vi "Paths to Commands.vi"(5 "Offset":cluster{"X Offset":dbl, "Y Offset":dbl}, 7 "Scaling":T1={"X Scaling (%)"=100.0, "Y Scaling (%)"=100.0}, 8 "error in (no error)":errorcluster, 10 "Path Properties":T3(array[cluster])=[{"Speed"=100.0, "Direction"=0, "Orientation (For Filled)"=enum."Vertical", "Max Spacing Between\nLines (For Filled)"=0.05, "Start and End Voltage"={"End Voltage"=0.0, "Start Voltage"=0.0}}, {"Speed"=100.0, "Direction"=0, "Orientation (For Filled)"=enum."Vertical", "Max Spacing Between\nLines (For Filled)"=0.05, "Start and End Voltage"={"End Voltage"=0.0, "Start Voltage"=0.0}}, {"Speed"=100.0, "Direction"=0, "Orientation (For Filled)"=enum."Vertical", "Max Spacing Between\nLines (For Filled)"=0.05, "Start and End Voltage"={"End Voltage"=0.0, "Start Voltage"=0.0}}, {"Speed"=100.0, "Direction"=0, "Orientation (For Filled)"=enum."Vertical", "Max Spacing Between\nLines (For Filled)"=0.05, "Start and End Voltage"={"End Voltage"=0.0, "Start Voltage"=0.0}}, {"Speed"=100.0, "Direction"=0, "Orientation (For Filled)"=enum."Vertical", "Max Spacing Between\nLines (For Filled)"=0.05, "Start and End Voltage"={"End Voltage"=0.0, "Start Voltage"=0.0}}, {"Speed"=100.0, "Direction"=0, "Orientation (For Filled)"=enum."Vertical", "Max Spacing Between\nLines (For Filled)"=0.05, "Start and End Voltage"={"End Voltage"=0.0, "Start Voltage"=0.0}}, {"Speed"=100.0, "Direction"=0, "Orientation (For Filled)"=enum."Vertical", "Max Spacing Between\nLines (For Filled)"=0.05, "Start and End Voltage"={"End Voltage"=0.0, "Start Voltage"=0.0}}, {"Speed"=100.0, "Direction"=0, "Orientation (For Filled)"=enum."Vertical", "Max Spacing Between\nLines (For Filled)"=0.05, "Start and End Voltage"={"End Voltage"=0.0, "Start Voltage"=0.0}}, {"Speed"=100.0, "Direction"=0, "Orientation (For Filled)"=enum."Vertical", "Max Spacing Between\nLines (For Filled)"=0.05, "Start and End Voltage"={"End Voltage"=0.0, "Start Voltage"=0.0}}, {"Speed"=100.0, "Direction"=0, "Orientation (For Filled)"=enum."Vertical", "Max Spacing Between\nLines (For Filled)"=0.05, "Start and End Voltage"={"End Voltage"=0.0, "Start Voltage"=0.0}}, {"Speed"=100.0, "Direction"=0, "Orientation (For Filled)"=enum."Vertical", "Max Spacing Between\nLines (For Filled)"=0.05, "Start and End Voltage"={"End Voltage"=0.0, "Start Voltage"=0.0}}, {"Speed"=100.0, "Direction"=0, "Orientation (For Filled)"=enum."Vertical", "Max Spacing Between\nLines (For Filled)"=0.05, "Start and End Voltage"={"End Voltage"=0.0, "Start Voltage"=0.0}}, {"Speed"=100.0, "Direction"=0, "Orientation (For Filled)"=enum."Vertical", "Max Spacing Between\nLines (For Filled)"=0.05, "Start and End Voltage"={"End Voltage"=0.0, "Start Voltage"=0.0}}, {"Speed"=100.0, "Direction"=0, "Orientation (For Filled)"=enum."Vertical", "Max Spacing Between\nLines (For Filled)"=0.05, "Start and End Voltage"={"End Voltage"=0.0, "Start Voltage"=0.0}}, {"Speed"=100.0, "Direction"=0, "Orientation (For Filled)"=enum."Vertical", "Max Spacing Between\nLines (For Filled)"=0.05, "Start and End Voltage"={"End Voltage"=0.0, "Start Voltage"=0.0}}, {"Speed"=100.0, "Direction"=0, "Orientation (For Filled)"=enum."Vertical", "Max Spacing Between\nLines (For Filled)"=0.05, "Start and End Voltage"={"End Voltage"=0.0, "Start Voltage"=0.0}}, {"Speed"=100.0, "Direction"=0, "Orientation (For Filled)"=enum."Vertical", "Max Spacing Between\nLines (For Filled)"=0.05, "Start and End Voltage"={"End Voltage"=0.0, "Start Voltage"=0.0}}, {"Speed"=100.0, "Direction"=0, "Orientation (For Filled)"=enum."Vertical", "Max Spacing Between\nLines (For Filled)"=0.05, "Start and End Voltage"={"End Voltage"=0.0, "Start Voltage"=0.0}}, {"Speed"=100.0, "Direction"=0, "Orientation (For Filled)"=enum."Vertical", "Max Spacing Between\nLines (For Filled)"=0.05, "Start and End Voltage"={"End Voltage"=0.0, "Start Voltage"=0.0}}, {"Speed"=100.0, "Direction"=0, "Orientation (For Filled)"=enum."Vertical", "Max Spacing Between\nLines (For Filled)"=0.05, "Start and End Voltage"={"End Voltage"=0.0, "Start Voltage"=0.0}}, {"Speed"=100.0, "Direction"=0, "Orientation (For Filled)"=enum."Vertical", "Max Spacing Between\nLines (For Filled)"=0.05, "Start and End Voltage"={"End Voltage"=0.0, "Start Voltage"=0.0}}, {"Speed"=100.0, "Direction"=0, "Orientation (For Filled)"=enum."Vertical", "Max Spacing Between\nLines (For Filled)"=0.05, "Start and End Voltage"={"End Voltage"=0.0, "Start Voltage"=0.0}}, {"Speed"=100.0, "Direction"=0, "Orientation (For Filled)"=enum."Vertical", "Max Spacing Between\nLines (For Filled)"=0.05, "Start and End Voltage"={"End Voltage"=0.0, "Start Voltage"=0.0}}, {"Speed"=100.0, "Direction"=0, "Orientation (For Filled)"=enum."Vertical", "Max Spacing Between\nLines (For Filled)"=0.05, "Start and End Voltage"={"End Voltage"=0.0, "Start Voltage"=0.0}}, {"Speed"=100.0, "Direction"=0, "Orientation (For Filled)"=enum."Vertical", "Max Spacing Between\nLines (For Filled)"=0.05, "Start and End Voltage"={"End Voltage"=0.0, "Start Voltage"=0.0}}, {"Speed"=100.0, "Direction"=0, "Orientation (For Filled)"=enum."Vertical", "Max Spacing Between\nLines (For Filled)"=0.05, "Start and End Voltage"={"End Voltage"=0.0, "Start Voltage"=0.0}}, {"Speed"=100.0, "Direction"=0, "Orientation (For Filled)"=enum."Vertical", "Max Spacing Between\nLines (For Filled)"=0.05, "Start and End Voltage"={"End Voltage"=0.0, "Start Voltage"=0.0}}, {"Speed"=100.0, "Direction"=0, "Orientation (For Filled)"=enum."Vertical", "Max Spacing Between\nLines (For Filled)"=0.05, "Start and End Voltage"={"End Voltage"=0.0, "Start Voltage"=0.0}}, {"Speed"=100.0, "Direction"=0, "Orientation (For Filled)"=enum."Vertical", "Max Spacing Between\nLines (For Filled)"=0.05, "Start and End Voltage"={"End Voltage"=0.0, "Start Voltage"=0.0}}, {"Speed"=100.0, "Direction"=0, "Orientation (For Filled)"=enum."Vertical", "Max Spacing Between\nLines (For Filled)"=0.05, "Start and End Voltage"={"End Voltage"=0.0, "Start Voltage"=0.0}}, {"Speed"=100.0, "Direction"=0, "Orientation (For Filled)"=enum."Vertical", "Max Spacing Between\nLines (For Filled)"=0.05, "Start and End Voltage"={"End Voltage"=0.0, "Start Voltage"=0.0}}, {"Speed"=100.0, "Direction"=0, "Orientation (For Filled)"=enum."Vertical", "Max Spacing Between\nLines (For Filled)"=0.05, "Start and End Voltage"={"End Voltage"=0.0, "Start Voltage"=0.0}}, {"Speed"=100.0, "Direction"=0, "Orientation (For Filled)"=enum."Vertical", "Max Spacing Between\nLines (For Filled)"=0.05, "Start and End Voltage"={"End Voltage"=0.0, "Start Voltage"=0.0}}, {"Speed"=100.0, "Direction"=0, "Orientation (For Filled)"=enum."Vertical", "Max Spacing Between\nLines (For Filled)"=0.05, "Start and End Voltage"={"End Voltage"=0.0, "Start Voltage"=0.0}}, {"Speed"=100.0, "Direction"=0, "Orientation (For Filled)"=enum."Vertical", "Max Spacing Between\nLines (For Filled)"=0.05, "Start and End Voltage"={"End Voltage"=0.0, "Start Voltage"=0.0}}, {"Speed"=100.0, "Direction"=0, "Orientation (For Filled)"=enum."Vertical", "Max Spacing Between\nLines (For Filled)"=0.05, "Start and End Voltage"={"End Voltage"=0.0, "Start Voltage"=0.0}}, {"Speed"=100.0, "Direction"=0, "Orientation (For Filled)"=enum."Vertical", "Max Spacing Between\nLines (For Filled)"=0.05, "Start and End Voltage"={"End Voltage"=0.0, "Start Voltage"=0.0}}, {"Speed"=100.0, "Direction"=0, "Orientation (For Filled)"=enum."Vertical", "Max Spacing Between\nLines (For Filled)"=0.05, "Start and End Voltage"={"End Voltage"=0.0, "Start Voltage"=0.0}}, {"Speed"=100.0, "Direction"=0, "Orientation (For Filled)"=enum."Vertical", "Max Spacing Between\nLines (For Filled)"=0.05, "Start and End Voltage"={"End Voltage"=0.0, "Start Voltage"=0.0}}, {"Speed"=100.0, "Direction"=0, "Orientation (For Filled)"=enum."Vertical", "Max Spacing Between\nLines (For Filled)"=0.05, "Start and End Voltage"={"End Voltage"=0.0, "Start Voltage"=0.0}}, {"Speed"=100.0, "Direction"=0, "Orientation (For Filled)"=enum."Vertical", "Max Spacing Between\nLines (For Filled)"=0.05, "Start and End Voltage"={"End Voltage"=0.0, "Start Voltage"=0.0}}, {"Speed"=100.0, "Direction"=0, "Orientation (For Filled)"=enum."Vertical", "Max Spacing Between\nLines (For Filled)"=0.05, "Start and End Voltage"={"End Voltage"=0.0, "Start Voltage"=0.0}}, {"Speed"=100.0, "Direction"=0, "Orientation (For Filled)"=enum."Vertical", "Max Spacing Between\nLines (For Filled)"=0.05, "Start and End Voltage"={"End Voltage"=0.0, "Start Voltage"=0.0}}, {"Speed"=100.0, "Direction"=0, "Orientation (For Filled)"=enum."Vertical", "Max Spacing Between\nLines (For Filled)"=0.05, "Start and End Voltage"={"End Voltage"=0.0, "Start Voltage"=0.0}}, {"Speed"=100.0, "Direction"=0, "Orientation (For Filled)"=enum."Vertical", "Max Spacing Between\nLines (For Filled)"=0.05, "Start and End Voltage"={"End Voltage"=0.0, "Start Voltage"=0.0}}, {"Speed"=100.0, "Direction"=0, "Orientation (For Filled)"=enum."Vertical", "Max Spacing Between\nLines (For Filled)"=0.05, "Start and End Voltage"={"End Voltage"=0.0, "Start Voltage"=0.0}}, {"Speed"=100.0, "Direction"=0, "Orientation (For Filled)"=enum."Vertical", "Max Spacing Between\nLines (For Filled)"=0.05, "Start and End Voltage"={"End Voltage"=0.0, "Start Voltage"=0.0}}, {"Speed"=100.0, "Direction"=0, "Orientation (For Filled)"=enum."Vertical", "Max Spacing Between\nLines (For Filled)"=0.05, "Start and End Voltage"={"End Voltage"=0.0, "Start Voltage"=0.0}}, {"Speed"=100.0, "Direction"=0, "Orientation (For Filled)"=enum."Vertical", "Max Spacing Between\nLines (For Filled)"=0.05, "Start and End Voltage"={"End Voltage"=0.0, "Start Voltage"=0.0}}, {"Speed"=100.0, "Direction"=0, "Orientation (For Filled)"=enum."Vertical", "Max Spacing Between\nLines (For Filled)"=0.05, "Start and End Voltage"={"End Voltage"=0.0, "Start Voltage"=0.0}}, {"Speed"=100.0, "Direction"=0, "Orientation (For Filled)"=enum."Vertical", "Max Spacing Between\nLines (For Filled)"=0.05, "Start and End Voltage"={"End Voltage"=0.0, "Start Voltage"=0.0}}, {"Speed"=100.0, "Direction"=0, "Orientation (For Filled)"=enum."Vertical", "Max Spacing Between\nLines (For Filled)"=0.05, "Start and End Voltage"={"End Voltage"=0.0, "Start Voltage"=0.0}}, {"Speed"=100.0, "Direction"=0, "Orientation (For Filled)"=enum."Vertical", "Max Spacing Between\nLines (For Filled)"=0.05, "Start and End Voltage"={"End Voltage"=0.0, "Start Voltage"=0.0}}, {"Speed"=100.0, "Direction"=0, "Orientation (For Filled)"=enum."Vertical", "Max Spacing Between\nLines (For Filled)"=0.05, "Start and End Voltage"={"End Voltage"=0.0, "Start Voltage"=0.0}}, {"Speed"=100.0, "Direction"=0, "Orientation (For Filled)"=enum."Vertical", "Max Spacing Between\nLines (For Filled)"=0.05, "Start and End Voltage"={"End Voltage"=0.0, "Start Voltage"=0.0}}, {"Speed"=100.0, "Direction"=0, "Orientation (For Filled)"=enum."Vertical", "Max Spacing Between\nLines (For Filled)"=0.05, "Start and End Voltage"={"End Voltage"=0.0, "Start Voltage"=0.0}}, {"Speed"=100.0, "Direction"=0, "Orientation (For Filled)"=enum."Vertical", "Max Spacing Between\nLines (For Filled)"=0.05, "Start and End Voltage"={"End Voltage"=0.0, "Start Voltage"=0.0}}, {"Speed"=100.0, "Direction"=0, "Orientation (For Filled)"=enum."Vertical", "Max Spacing Between\nLines (For Filled)"=0.05, "Start and End Voltage"={"End Voltage"=0.0, "Start Voltage"=0.0}}, {"Speed"=100.0, "Direction"=0, "Orientation (For Filled)"=enum."Vertical", "Max Spacing Between\nLines (For Filled)"=0.05, "Start and End Voltage"={"End Voltage"=0.0, "Start Voltage"=0.0}}, {"Speed"=100.0, "Direction"=0, "Orientation (For Filled)"=enum."Vertical", "Max Spacing Between\nLines (For Filled)"=0.05, "Start and End Voltage"={"End Voltage"=0.0, "Start Voltage"=0.0}}, {"Speed"=100.0, "Direction"=0, "Orientation (For Filled)"=enum."Vertical", "Max Spacing Between\nLines (For Filled)"=0.05, "Start and End Voltage"={"End Voltage"=0.0, "Start Voltage"=0.0}}, {"Speed"=100.0, "Direction"=0, "Orientation (For Filled)"=enum."Vertical", "Max Spacing Between\nLines (For Filled)"=0.05, "Start and End Voltage"={"End Voltage"=0.0, "Start Voltage"=0.0}}, {"Speed"=100.0, "Direction"=0, "Orientation (For Filled)"=enum."Vertical", "Max Spacing Between\nLines (For Filled)"=0.05, "Start and End Voltage"={"End Voltage"=0.0, "Start Voltage"=0.0}}, {"Speed"=100.0, "Direction"=0, "Orientation (For Filled)"=enum."Vertical", "Max Spacing Between\nLines (For Filled)"=0.05, "Start and End Voltage"={"End Voltage"=0.0, "Start Voltage"=0.0}}, {"Speed"=100.0, "Direction"=0, "Orientation (For Filled)"=enum."Vertical", "Max Spacing Between\nLines (For Filled)"=0.05, "Start and End Voltage"={"End Voltage"=0.0, "Start Voltage"=0.0}}, {"Speed"=100.0, "Direction"=0, "Orientation (For Filled)"=enum."Vertical", "Max Spacing Between\nLines (For Filled)"=0.05, "Start and End Voltage"={"End Voltage"=0.0, "Start Voltage"=0.0}}, {"Speed"=100.0, "Direction"=0, "Orientation (For Filled)"=enum."Vertical", "Max Spacing Between\nLines (For Filled)"=0.05, "Start and End Voltage"={"End Voltage"=0.0, "Start Voltage"=0.0}}, {"Speed"=100.0, "Direction"=0, "Orientation (For Filled)"=enum."Vertical", "Max Spacing Between\nLines (For Filled)"=0.05, "Start and End Voltage"={"End Voltage"=0.0, "Start Voltage"=0.0}}, {"Speed"=100.0, "Direction"=0, "Orientation (For Filled)"=enum."Vertical", "Max Spacing Between\nLines (For Filled)"=0.05, "Start and End Voltage"={"End Voltage"=0.0, "Start Voltage"=0.0}}, {"Speed"=100.0, "Direction"=0, "Orientation (For Filled)"=enum."Vertical", "Max Spacing Between\nLines (For Filled)"=0.05, "Start and End Voltage"={"End Voltage"=0.0, "Start Voltage"=0.0}}, {"Speed"=100.0, "Direction"=0, "Orientation (For Filled)"=enum."Vertical", "Max Spacing Between\nLines (For Filled)"=0.05, "Start and End Voltage"={"End Voltage"=0.0, "Start Voltage"=0.0}}, {"Speed"=100.0, "Direction"=0, "Orientation (For Filled)"=enum."Vertical", "Max Spacing Between\nLines (For Filled)"=0.05, "Start and End Voltage"={"End Voltage"=0.0, "Start Voltage"=0.0}}, {"Speed"=100.0, "Direction"=0, "Orientation (For Filled)"=enum."Vertical", "Max Spacing Between\nLines (For Filled)"=0.05, "Start and End Voltage"={"End Voltage"=0.0, "Start Voltage"=0.0}}, {"Speed"=100.0, "Direction"=0, "Orientation (For Filled)"=enum."Vertical", "Max Spacing Between\nLines (For Filled)"=0.05, "Start and End Voltage"={"End Voltage"=0.0, "Start Voltage"=0.0}}, {"Speed"=100.0, "Direction"=0, "Orientation (For Filled)"=enum."Vertical", "Max Spacing Between\nLines (For Filled)"=0.05, "Start and End Voltage"={"End Voltage"=0.0, "Start Voltage"=0.0}}, {"Speed"=100.0, "Direction"=0, "Orientation (For Filled)"=enum."Vertical", "Max Spacing Between\nLines (For Filled)"=0.05, "Start and End Voltage"={"End Voltage"=0.0, "Start Voltage"=0.0}}, {"Speed"=100.0, "Direction"=0, "Orientation (For Filled)"=enum."Vertical", "Max Spacing Between\nLines (For Filled)"=0.05, "Start and End Voltage"={"End Voltage"=0.0, "Start Voltage"=0.0}}, {"Speed"=100.0, "Direction"=0, "Orientation (For Filled)"=enum."Vertical", "Max Spacing Between\nLines (For Filled)"=0.05, "Start and End Voltage"={"End Voltage"=0.0, "Start Voltage"=0.0}}, {"Speed"=100.0, "Direction"=0, "Orientation (For Filled)"=enum."Vertical", "Max Spacing Between\nLines (For Filled)"=0.05, "Start and End Voltage"={"End Voltage"=0.0, "Start Voltage"=0.0}}, {"Speed"=100.0, "Direction"=0, "Orientation (For Filled)"=enum."Vertical", "Max Spacing Between\nLines (For Filled)"=0.05, "Start and End Voltage"={"End Voltage"=0.0, "Start Voltage"=0.0}}, {"Speed"=100.0, "Direction"=0, "Orientation (For Filled)"=enum."Vertical", "Max Spacing Between\nLines (For Filled)"=0.05, "Start and End Voltage"={"End Voltage"=0.0, "Start Voltage"=0.0}}, {"Speed"=100.0, "Direction"=0, "Orientation (For Filled)"=enum."Vertical", "Max Spacing Between\nLines (For Filled)"=0.05, "Start and End Voltage"={"End Voltage"=0.0, "Start Voltage"=0.0}}, {"Speed"=100.0, "Direction"=0, "Orientation (For Filled)"=enum."Vertical", "Max Spacing Between\nLines (For Filled)"=0.05, "Start and End Voltage"={"End Voltage"=0.0, "Start Voltage"=0.0}}, {"Speed"=100.0, "Direction"=0, "Orientation (For Filled)"=enum."Vertical", "Max Spacing Between\nLines (For Filled)"=0.05, "Start and End Voltage"={"End Voltage"=0.0, "Start Voltage"=0.0}}, {"Speed"=100.0, "Direction"=0, "Orientation (For Filled)"=enum."Vertical", "Max Spacing Between\nLines (For Filled)"=0.05, "Start and End Voltage"={"End Voltage"=0.0, "Start Voltage"=0.0}}, {"Speed"=100.0, "Direction"=0, "Orientation (For Filled)"=enum."Vertical", "Max Spacing Between\nLines (For Filled)"=0.05, "Start and End Voltage"={"End Voltage"=0.0, "Start Voltage"=0.0}}, {"Speed"=100.0, "Direction"=0, "Orientation (For Filled)"=enum."Vertical", "Max Spacing Between\nLines (For Filled)"=0.05, "Start and End Voltage"={"End Voltage"=0.0, "Start Voltage"=0.0}}, {"Speed"=100.0, "Direction"=0, "Orientation (For Filled)"=enum."Vertical", "Max Spacing Between\nLines (For Filled)"=0.05, "Start and End Voltage"={"End Voltage"=0.0, "Start Voltage"=0.0}}, {"Speed"=100.0, "Direction"=0, "Orientation (For Filled)"=enum."Vertical", "Max Spacing Between\nLines (For Filled)"=0.05, "Start and End Voltage"={"End Voltage"=0.0, "Start Voltage"=0.0}}, {"Speed"=100.0, "Direction"=0, "Orientation (For Filled)"=enum."Vertical", "Max Spacing Between\nLines (For Filled)"=0.05, "Start and End Voltage"={"End Voltage"=0.0, "Start Voltage"=0.0}}, {"Speed"=100.0, "Direction"=0, "Orientation (For Filled)"=enum."Vertical", "Max Spacing Between\nLines (For Filled)"=0.05, "Start and End Voltage"={"End Voltage"=0.0, "Start Voltage"=0.0}}, {"Speed"=100.0, "Direction"=0, "Orientation (For Filled)"=enum."Vertical", "Max Spacing Between\nLines (For Filled)"=0.05, "Start and End Voltage"={"End Voltage"=0.0, "Start Voltage"=0.0}}, {"Speed"=100.0, "Direction"=0, "Orientation (For Filled)"=enum."Vertical", "Max Spacing Between\nLines (For Filled)"=0.05, "Start and End Voltage"={"End Voltage"=0.0, "Start Voltage"=0.0}}, {"Speed"=100.0, "Direction"=0, "Orientation (For Filled)"=enum."Vertical", "Max Spacing Between\nLines (For Filled)"=0.05, "Start and End Voltage"={"End Voltage"=0.0, "Start Voltage"=0.0}}, {"Speed"=100.0, "Direction"=0, "Orientation (For Filled)"=enum."Vertical", "Max Spacing Between\nLines (For Filled)"=0.05, "Start and End Voltage"={"End Voltage"=0.0, "Start Voltage"=0.0}}, {"Speed"=100.0, "Direction"=0, "Orientation (For Filled)"=enum."Vertical", "Max Spacing Between\nLines (For Filled)"=0.05, "Start and End Voltage"={"End Voltage"=0.0, "Start Voltage"=0.0}}, {"Speed"=100.0, "Direction"=0, "Orientation (For Filled)"=enum."Vertical", "Max Spacing Between\nLines (For Filled)"=0.05, "Start and End Voltage"={"End Voltage"=0.0, "Start Voltage"=0.0}}, {"Speed"=100.0, "Direction"=0, "Orientation (For Filled)"=enum."Vertical", "Max Spacing Between\nLines (For Filled)"=0.05, "Start and End Voltage"={"End Voltage"=0.0, "Start Voltage"=0.0}}, {"Speed"=100.0, "Direction"=0, "Orientation (For Filled)"=enum."Vertical", "Max Spacing Between\nLines (For Filled)"=0.05, "Start and End Voltage"={"End Voltage"=0.0, "Start Voltage"=0.0}}, {"Speed"=100.0, "Direction"=0, "Orientation (For Filled)"=enum."Vertical", "Max Spacing Between\nLines (For Filled)"=0.05, "Start and End Voltage"={"End Voltage"=0.0, "Start Voltage"=0.0}}, {"Speed"=100.0, "Direction"=0, "Orientation (For Filled)"=enum."Vertical", "Max Spacing Between\nLines (For Filled)"=0.05, "Start and End Voltage"={"End Voltage"=0.0, "Start Voltage"=0.0}}] {"Direction" items=["Forward", "Backward"]}, 11 "paths":T5(array[cluster])) -> (0 "error out":errorcluster, 3 "Lithography Information":T2(array[cluster]))   [LabVIEW 2011]
doc: "This VI processes the rectangles' data and outputs lithography data."
uses:
  <vilib>/Analysis/Matrix/Datatypes/RealMatrix.ctl
  <vilib>/Analysis/Matrix/NI_Matrix.lvlib
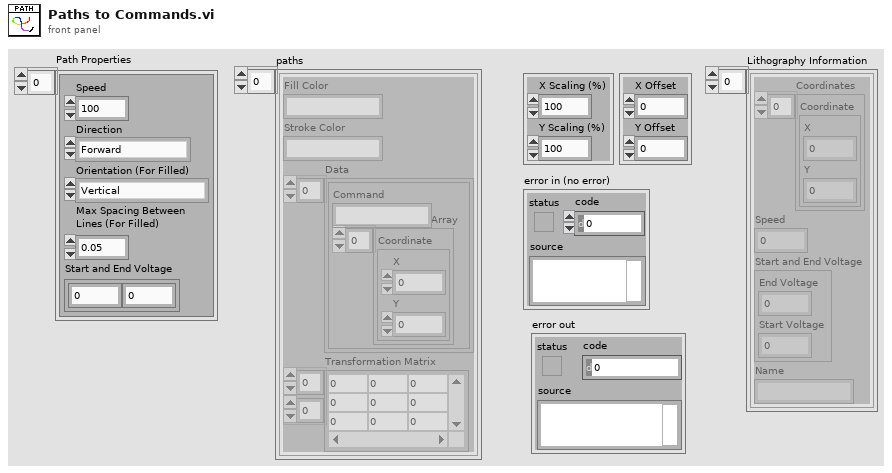
[diagram p1: front panel]
types:
  T1 = cluster{"X Scaling (%)":dbl, "Y Scaling (%)":dbl}
  T2 = cluster{"Coordinates":cluster{"X":dbl, "Y":dbl}[], "Speed":dbl, "Start and End Voltage":cluster{"End Voltage":dbl, "Start Voltage":dbl}, "Name":string}[]
  T3 = cluster{"Speed":dbl, "Direction":u16, "Orientation (For Filled)":enum16{"Horizontal", "Vertical"}, "Max Spacing Between\nLines (For Filled)":dbl, "Start and End Voltage":cluster{"End Voltage":dbl, "Start Voltage":dbl}}[]
  T4 = typedef "NI_Matrix.lvlib/RealMatrix.ctl" = dbl[][]
  T5 = cluster{"Fill Color":string, "Stroke Color":string, "Data":cluster{"Command":string, "Coordinate Array":cluster{"X":dbl, "Y":dbl}[]}[], "Transformation Matrix":T4}[]
  T6 = cluster{"Command":string, "Coordinate Array":cluster{"X":dbl, "Y":dbl}[]}[]
  T7 = cluster{cluster{dbl, dbl}[], "Speed":dbl, "Start and End Voltage":cluster{"End Voltage":dbl, "Start Voltage":dbl}, string}
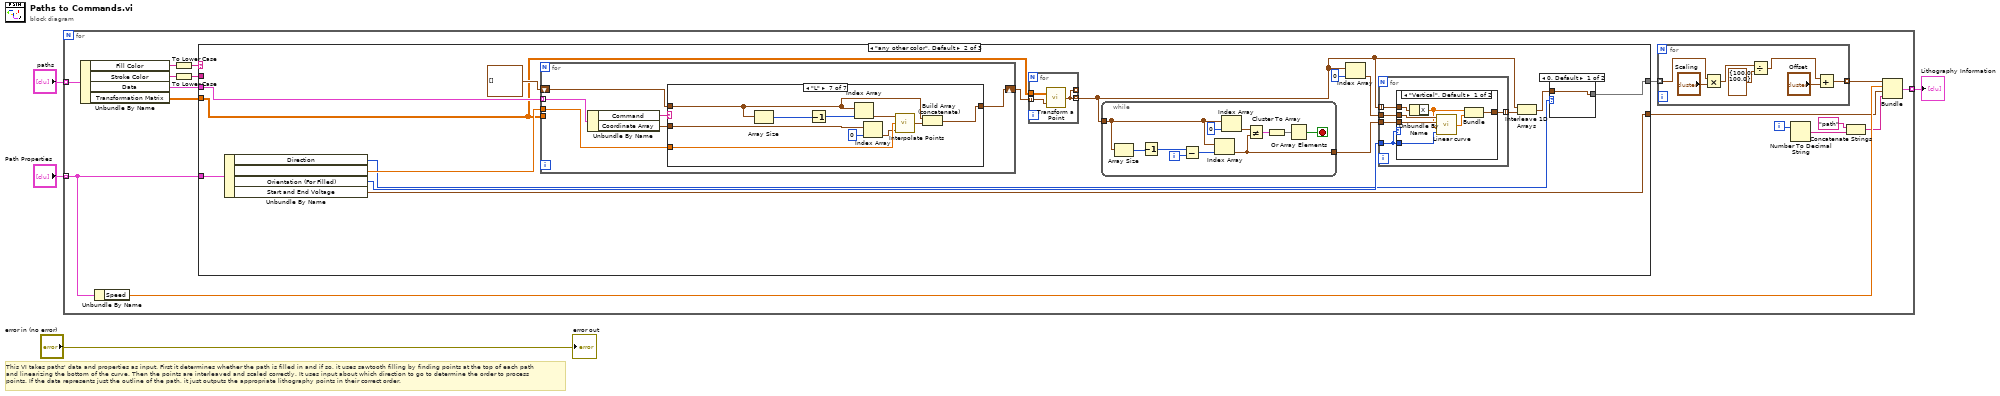
[diagram p0: block diagram]
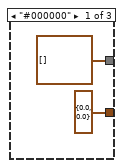
[diagram p2: hidden frame]
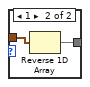
[diagram p3: hidden frame]
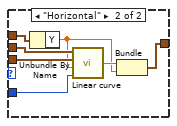
[diagram p4: hidden frame]
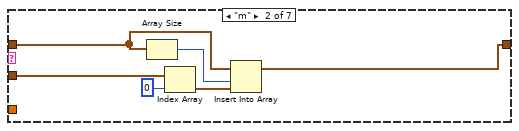
[diagram p6: hidden frame]
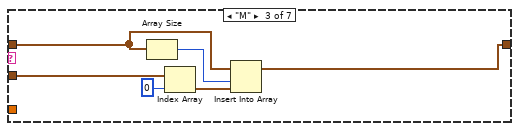
[diagram p7: hidden frame]
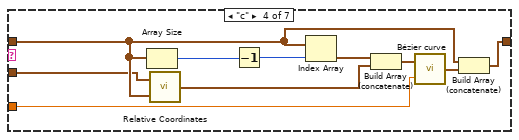
[diagram p8: hidden frame]
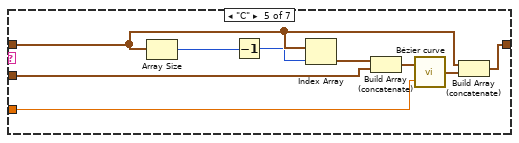
[diagram p9: hidden frame]
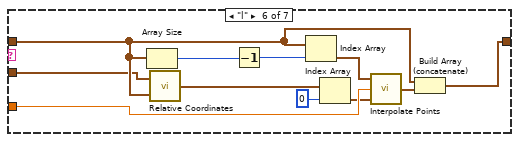
[diagram p10: hidden frame]
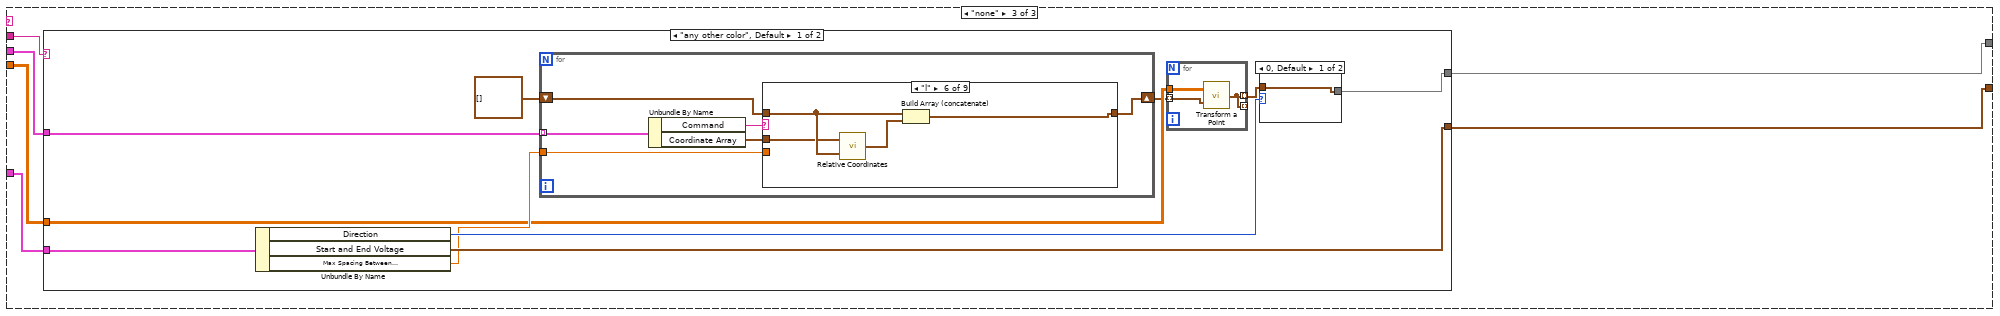
[diagram p11: hidden frame]
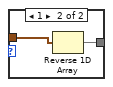
[diagram p12: hidden frame]
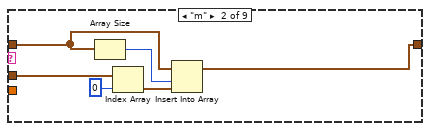
[diagram p14: hidden frame]
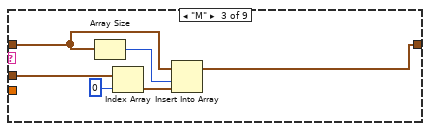
[diagram p15: hidden frame]
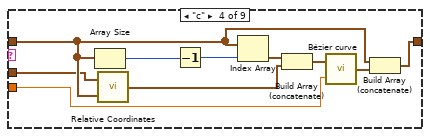
[diagram p16: hidden frame]
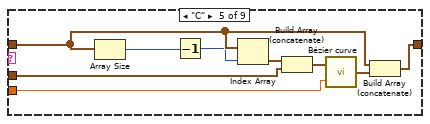
[diagram p17: hidden frame]
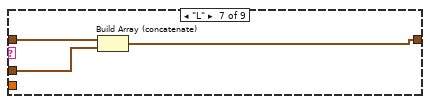
[diagram p18: hidden frame]
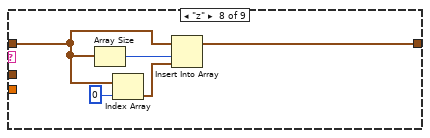
[diagram p19: hidden frame]
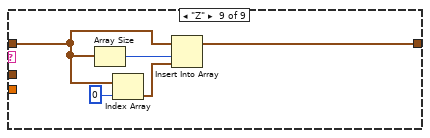
[diagram p20: hidden frame]
diagram:
  # "This VI takes paths' data and properties as input. First it determines whether the path is filled in and if so, it uses sawtooth filling by finding points at the top of each path \nand linearizing the bottom of the curve. Then the points are interleaved and scaled correctly. It uses input about which direction to go to determine the order to process \npoints. If the data represents just the outline of the path, it just outputs the appropriate lithography points in their correct order."
  n1 = for {
    tunnel: "paths" -> [w14] mode=indexing
    tunnel: "Path Properties" -> [w16] mode=indexing
    tunnel: [w17] -> w1 mode=indexing
    i -> [w8]
    n2 = Unbundle By Name(w14) -> ("Fill Color"=w21:string, "Stroke Color"=w19:string, "Data"=w13:T6, "Transformation Matrix"=w5:T4)
    n3 = Unbundle By Name(w16) -> ("Speed"=w15:dbl)
    n4 = To Lower Case(string=w21) -> (all lower case string=w20:string)
    n5 = To Lower Case(string=w19) -> (all lower case string=w18:string)
    n6 = case shown="\"any other color\", Default" w20 {
      tunnel: w18 -> [_ _ w143]
      tunnel: w16 -> [_ w45 w146]
      tunnel: [cluster{"X":dbl, "Y":dbl}[] [] w37 w145] -> w7
      tunnel: w13 -> [_ w35 w147]
      tunnel: w5 -> [_ w31 w144]
      tunnel: [cluster{"End Voltage":dbl, "Start Voltage":dbl} {"End Voltage"=0.0, "Start Voltage"=0.0} ("Start and End Voltage") w34 w142] -> w12
      frame "#000000" {
      }
      frame "any other color", Default {
        n7 = Unbundle By Name(w45) -> ("Direction"=w36:u16, "Max Spacing Between\nLines (For Filled)"=w39:dbl, "Orientation (For Filled)"=w43:enum16{"Horizontal", "Vertical"}, "Start and End Voltage"=w34:cluster{"End Voltage":dbl, "Start Voltage":dbl})
        n8 = for {
          tunnel: w35 -> [w88] mode=indexing
          shift-right: [w84] -> w33
          shift-left: cluster{"X":dbl, "Y":dbl}[] [] -> [w86]
          tunnel: w39 -> [w85]
          tunnel: w31 -> [_]
          n9 = Unbundle By Name(w88) -> ("Command"=w87:string, "Coordinate Array"=w83:cluster{"X":dbl, "Y":dbl}[])
          n10 = case shown="\"L\"" w87 {
            tunnel: w83 -> [_ w90 w96 w102 w112 w121 w132]
            tunnel: w86 -> [w89 w92 w97 w110 w119 w123 w133]
            tunnel: [w89 w93 w98 w104 w114 w129 w140] -> w84
            tunnel: w85 -> [_ _ _ w103 w113 w130 w141]
            frame "other letters", Default {
            }
            frame "m" {
              n11 = Array Size(array=w92) -> (size(s)=w95:i32)
              n12 = Index Array(array=w90, index=0) -> (element=w94:cluster{"X":dbl, "Y":dbl})
              n13 = Insert Into Array(array=w92, index=w95, new element=w94) -> (w93:cluster{"X":dbl, "Y":dbl}[])
            }
            frame "M" {
              n14 = Array Size(array=w97) -> (size(s)=w100:i32)
              n15 = Index Array(array=w96, index=0) -> (element=w99:cluster{"X":dbl, "Y":dbl})
              n16 = Insert Into Array(array=w97, index=w100, new element=w99) -> (w98:cluster{"X":dbl, "Y":dbl}[])
            }
            frame "c" {
              n17 = Array Size(array=w110) -> (size(s)=w106:i32)
              n18 = call "Relative Coordinates.vi"("All Coordinates"=w110, "Command Coordinates"=w102) -> ("Adjusted Command Coordinates"=w108:cluster{"X":dbl, "Y":dbl}[])
              n19 = Decrement(x=w106) -> (x-1=w105:i32)
              n20 = Index Array(array=w110, index=w105) -> (element=w109:cluster{"X":dbl, "Y":dbl})
              n21 = Build Array (concatenate)(w109, w108) -> (w107:cluster{"X":dbl, "Y":dbl}[])
              n22 = call "Bézier curve.vi"("Spacing"=w103, "Parameters"=w107) -> ("Coordinate Array"=w111:cluster{"X":dbl, "Y":dbl}[])
              n23 = Build Array (concatenate)(w110, w111) -> (w104:cluster{"X":dbl, "Y":dbl}[])
            }
            frame "C" {
              n24 = Array Size(array=w119) -> (size(s)=w116:i32)
              n25 = Decrement(x=w116) -> (x-1=w115:i32)
              n26 = Index Array(array=w119, index=w115) -> (element=w118:cluster{"X":dbl, "Y":dbl})
              n27 = Build Array (concatenate)(w118, w112) -> (w117:cluster{"X":dbl, "Y":dbl}[])
              n28 = call "Bézier curve.vi"("Spacing"=w113, "Parameters"=w117) -> ("Coordinate Array"=w120:cluster{"X":dbl, "Y":dbl}[])
              n29 = Build Array (concatenate)(w119, w120) -> (w114:cluster{"X":dbl, "Y":dbl}[])
            }
            frame "l" {
              n30 = Array Size(array=w123) -> (size(s)=w125:i32)
              n31 = call "Relative Coordinates.vi"("All Coordinates"=w123, "Command Coordinates"=w121) -> ("Adjusted Command Coordinates"=w128:cluster{"X":dbl, "Y":dbl}[])
              n32 = Decrement(x=w125) -> (x-1=w124:i32)
              n33 = Index Array(array=w123, index=w124) -> (element=w127:cluster{"X":dbl, "Y":dbl})
              n34 = Index Array(array=w128, index=0) -> (element=w126:cluster{"X":dbl, "Y":dbl})
              n35 = call "Interpolate Points.vi"("End Point"=w126, "Distance between Points"=w130, "Start Point"=w127) -> ("Output Point Array"=w131:cluster{"X":dbl, "Y":dbl}[])
              n36 = Build Array (concatenate)(w123, w131) -> (w129:cluster{"X":dbl, "Y":dbl}[])
            }
            frame "L" {
              n37 = Array Size(array=w133) -> (size(s)=w135:i32)
              n38 = Decrement(x=w135) -> (x-1=w134:i32)
              n39 = Index Array(array=w133, index=w134) -> (element=w138:cluster{"X":dbl, "Y":dbl})
              n40 = Index Array(array=w132, index=0) -> (element=w136:cluster{"X":dbl, "Y":dbl})
              n41 = call "Interpolate Points.vi"("End Point"=w136, "Distance between Points"=w141, "Start Point"=w138) -> ("Output Point Array"=w139:cluster{"X":dbl, "Y":dbl}[])
              n42 = Build Array (concatenate)(w133, w139) -> (w140:cluster{"X":dbl, "Y":dbl}[])
            }
          }
        }
        n43 = for {
          tunnel: [w47] -> w32 mode=indexing
          tunnel: w31 -> [w49]
          tunnel: w33 -> [w48] mode=indexing
          tunnel: [w47] -> _ mode=indexing
          n44 = call "Transform a Point.vi"("Point to Transform"=w48, "Transformation Matrix"=w49) -> ("Transformed Point"=w47:cluster{"X":dbl, "Y":dbl})
        }
        n45 = while {
          tunnel: w32 -> [w72]
          tunnel: [w73] -> w41
          i -> [w79]
          stop <- w75 stop-if-true
          n46 = Array Size(array=w72) -> (size(s)=w81:i32)
          n47 = Decrement(x=w81) -> (x-1=w80:i32)
          n48 = Subtract(x=w80, y=w79) -> (x-y=w78:i32)
          n49 = Index Array(array=w72, index=w78) -> (element=w73:cluster{"X":dbl, "Y":dbl})
          n50 = Index Array(array=w72, index=0) -> (element=w77:cluster{"X":dbl, "Y":dbl})
          n51 = Not Equal?(x=w77, y=w73) -> (x != y?=w76:cluster{"X":bool, "Y":bool})
          n52 = Cluster To Array(cluster=w76) -> (array=w74:bool[])
          n53 = Or Array Elements(Boolean array=w74) -> (logical OR=w75:bool)
        }
        n54 = Index Array(array=w32, index=0) -> (element=w42:cluster{"X":dbl, "Y":dbl})
        n55 = for {
          tunnel: w43 -> [w55]
          tunnel: w32 -> [w54] mode=indexing
          tunnel: w42 -> [w57]
          tunnel: w41 -> [w56]
          tunnel: [w53] -> w40 mode=indexing
          n56 = case shown="\"Vertical\", Default" w55 {
            tunnel: w57 -> [w64 w71]
            tunnel: w56 -> [w63 w70]
            tunnel: w55 -> [w62 w69]
            tunnel: w54 -> [w61 w68]
            tunnel: [w60 w67] -> w53
            frame "Vertical", Default {
              n57 = Unbundle By Name(w61) -> ("X"=w59:dbl)
              n58 = call "Linear curve.vi"("Orientation"=w62, "Input X or Y Value"=w59, "Point 2"=w63, "Point 1"=w64) -> ("Output Value"=w58:dbl)
              n59 = Bundle("X"=w59, "Output Value"=w58) -> (w60:cluster{"X":dbl, "Output Value":dbl})  [unwired: 1 in]
            }
            frame "Horizontal" {
              n60 = Unbundle By Name(w68) -> ("Y"=w65:dbl)
              n61 = call "Linear curve.vi"("Orientation"=w69, "Input X or Y Value"=w65, "Point 2"=w70, "Point 1"=w71) -> ("Output Value"=w66:dbl)
              n62 = Bundle("Output Value"=w66, "Y"=w65) -> (w67:cluster{"Output Value":dbl, "Y":dbl})  [unwired: 1 in]
            }
          }
        }
        n63 = Interleave 1D Arrays(w32, w40) -> (w38:cluster{"Output Value":dbl, "Y":dbl}[])
        n64 = case shown="0, Default" w36 {
          tunnel: [w50 w51] -> w37
          tunnel: w38 -> [w50 w52]
          frame 0, Default {
          }
          frame 1 {
            n65 = Reverse 1D Array(array=w52) -> (reversed array=w51:cluster{"Output Value":dbl, "Y":dbl}[])
          }
        }
      }
      frame "none" {
        n66 = case shown="\"any other color\", Default" w143 {
          tunnel: w147 -> [w157 _]
          tunnel: w146 -> [w155 _]
          tunnel: [w154 cluster{"X":dbl, "Y":dbl}[] []] -> w145
          tunnel: w144 -> [w150 _]
          tunnel: [w152 cluster{"End Voltage":dbl, "Start Voltage":dbl} {"End Voltage"=0.0, "Start Voltage"=0.0} ("Start and End Voltage")] -> w142
          frame "any other color", Default {
            n67 = Unbundle By Name(w155) -> ("Direction"=w153:u16, "Start and End Voltage"=w152:cluster{"End Voltage":dbl, "Start Voltage":dbl}, "Max Spacing Between\nLines (For Filled)"=w151:dbl)
            n68 = for {
              tunnel: w157 -> [w169] mode=indexing
              shift-right: [w165] -> w149
              shift-left: cluster{"X":dbl, "Y":dbl}[] [] -> [w166]
              tunnel: w151 -> [w164]
              n69 = Unbundle By Name(w169) -> ("Command"=w168:string, "Coordinate Array"=w167:cluster{"X":dbl, "Y":dbl}[])
              n70 = case shown="\"l\"" w168 {
                tunnel: w167 -> [_ w171 w177 w183 w193 w202 w206 _ _]
                tunnel: w166 -> [w170 w172 w178 w190 w199 w204 w208 w209 w214]
                tunnel: [w170 w173 w179 w192 w201 w203 w207 w210 w215] -> w165
                tunnel: w164 -> [_ _ _ w184 w194 _ _ _ _]
                frame "other letters", Default {
                }
                frame "m" {
                  n71 = Array Size(array=w172) -> (size(s)=w175:i32)
                  n72 = Index Array(array=w171, index=0) -> (element=w174:cluster{"X":dbl, "Y":dbl})
                  n73 = Insert Into Array(array=w172, index=w175, new element=w174) -> (w173:cluster{"X":dbl, "Y":dbl}[])
                }
                frame "M" {
                  n74 = Array Size(array=w178) -> (size(s)=w181:i32)
                  n75 = Index Array(array=w177, index=0) -> (element=w180:cluster{"X":dbl, "Y":dbl})
                  n76 = Insert Into Array(array=w178, index=w181, new element=w180) -> (w179:cluster{"X":dbl, "Y":dbl}[])
                }
                frame "c" {
                  n77 = Array Size(array=w190) -> (size(s)=w186:i32)
                  n78 = call "Relative Coordinates.vi"("All Coordinates"=w190, "Command Coordinates"=w183) -> ("Adjusted Command Coordinates"=w188:cluster{"X":dbl, "Y":dbl}[])
                  n79 = Decrement(x=w186) -> (x-1=w185:i32)
                  n80 = Index Array(array=w190, index=w185) -> (element=w189:cluster{"X":dbl, "Y":dbl})
                  n81 = Build Array (concatenate)(w189, w188) -> (w187:cluster{"X":dbl, "Y":dbl}[])
                  n82 = call "Bézier curve.vi"("Spacing"=w184, "Parameters"=w187) -> ("Coordinate Array"=w191:cluster{"X":dbl, "Y":dbl}[])
                  n83 = Build Array (concatenate)(w190, w191) -> (w192:cluster{"X":dbl, "Y":dbl}[])
                }
                frame "C" {
                  n84 = Array Size(array=w199) -> (size(s)=w196:i32)
                  n85 = Decrement(x=w196) -> (x-1=w195:i32)
                  n86 = Index Array(array=w199, index=w195) -> (element=w198:cluster{"X":dbl, "Y":dbl})
                  n87 = Build Array (concatenate)(w198, w193) -> (w197:cluster{"X":dbl, "Y":dbl}[])
                  n88 = call "Bézier curve.vi"("Spacing"=w194, "Parameters"=w197) -> ("Coordinate Array"=w200:cluster{"X":dbl, "Y":dbl}[])
                  n89 = Build Array (concatenate)(w199, w200) -> (w201:cluster{"X":dbl, "Y":dbl}[])
                }
                frame "l" {
                  n90 = call "Relative Coordinates.vi"("All Coordinates"=w204, "Command Coordinates"=w202) -> ("Adjusted Command Coordinates"=w205:cluster{"X":dbl, "Y":dbl}[])
                  n91 = Build Array (concatenate)(w204, w205) -> (w203:cluster{"X":dbl, "Y":dbl}[])
                }
                frame "L" {
                  n92 = Build Array (concatenate)(w208, w206) -> (w207:cluster{"X":dbl, "Y":dbl}[])
                }
                frame "z" {
                  n93 = Array Size(array=w209) -> (size(s)=w212:i32)
                  n94 = Index Array(array=w209, index=0) -> (element=w211:cluster{"X":dbl, "Y":dbl})
                  n95 = Insert Into Array(array=w209, index=w212, new element=w211) -> (w210:cluster{"X":dbl, "Y":dbl}[])
                }
                frame "Z" {
                  n96 = Array Size(array=w214) -> (size(s)=w217:i32)
                  n97 = Index Array(array=w214, index=0) -> (element=w216:cluster{"X":dbl, "Y":dbl})
                  n98 = Insert Into Array(array=w214, index=w217, new element=w216) -> (w215:cluster{"X":dbl, "Y":dbl}[])
                }
              }
            }
            n99 = for {
              tunnel: [w158] -> _ mode=indexing
              tunnel: w150 -> [w160]
              tunnel: w149 -> [w159] mode=indexing
              tunnel: [w158] -> w148 mode=indexing
              n100 = call "Transform a Point.vi"("Point to Transform"=w159, "Transformation Matrix"=w160) -> ("Transformed Point"=w158:cluster{"X":dbl, "Y":dbl})
            }
            n101 = case shown="0, Default" w153 {
              tunnel: [w161 w162] -> w154
              tunnel: w148 -> [w161 w163]
              frame 0, Default {
              }
              frame 1 {
                n102 = Reverse 1D Array(array=w163) -> (reversed array=w162:cluster{"X":dbl, "Y":dbl}[])
              }
            }
          }
          frame "#000000" {
          }
        }
      }
    }
    n103 = for {
      tunnel: w7 -> [w28] mode=indexing
      tunnel: [w22] -> w6 mode=indexing
      n104 = Multiply(x=w28, y="Scaling") -> (x*y=w26:cluster{dbl, dbl})
      n105 = Divide(x=w26, y=cluster{dbl, dbl} {100.0, 100.0}) -> (x/y=w24:cluster{dbl, dbl})
      n106 = Add(x=w24, y="Offset") -> (x+y=w22:cluster{dbl, dbl})
    }
    n107 = Number To Decimal String(number=w8) -> (decimal integer string=w10:string)  [unwired: 1 in]
    n108 = Concatenate Strings("path", w10) -> (w9:string)
    n109 = Bundle(w6, "Speed"=w15, "Start and End Voltage"=w12, w9) -> (w17:T7)  [unwired: 1 in]
  }
  "Lithography Information" <- w1
  "error out" <- "error in (no error)"
